vi "Write Section.vi"(8 "error in (no error)":errorcluster, 9 "Section Data":variant, 10 "Section Name":string, 11 "Configuration File in":refnum<class "Configuration File.lvclass">) -> (0 "error out":errorcluster, 3 "Configuration File out":refnum<class "Configuration File.lvclass">)   [LabVIEW 2019, in "Configuration File.lvlib" / "Configuration File.lvclass"]
doc: "This VI writes the variant's attributes in the section specified."
uses:
  Configuration File.lvclass
  Configuration File.lvclass/Configuration File.ctl
  <vilib>/Utility/config.llb/Write Key (String).vi
  <vilib>/Utility/config.llb/Write Key (Boolean).vi
  <vilib>/Utility/config.llb/Write Key (Double).vi
  <vilib>/Utility/config.llb/Write Key (U32).vi
  <vilib>/Utility/config.llb/Write Key (I32).vi
  <vilib>/Utility/config.llb/Write Key (Path).vi
  <vilib>/Utility/Data Type/NI_Data Type.lvlib
  <vilib>/Utility/config.llb/NI_LVConfig.lvlib
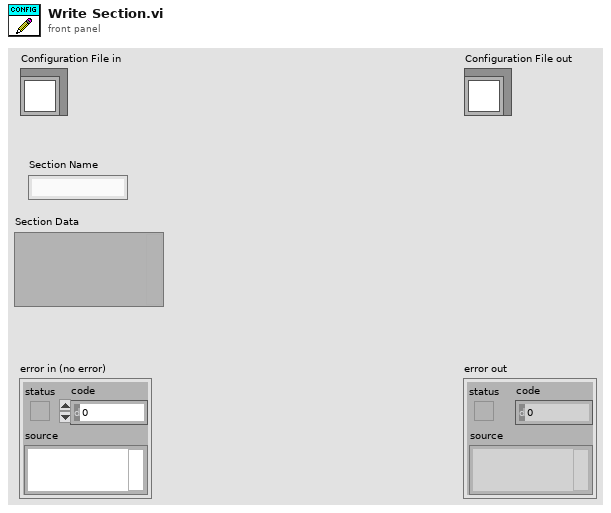
[diagram p1: front panel]
types:
  T1 = typedef "NI_LVConfig.lvlib/Config Data RefNum.ctl" = refnum<k1>
  T2 = typedef "NI_Data Type.lvlib/Data Type.ctl" = enum8{"Invalid Type", "Void", "I8", "I16", "I32", "I64", "U8", "U16", "U32", "U64", "Single Float", "Double Float", "Extended Float", "Single Complex", "Double Complex", "Extended Complex", "Enum U8", "Enum U16", "Enum U32", "Enum U64", "Single Float With Unit", "Double Float With Unit", "Extended Float With Unit", "Single Complex with Unit", "Double Complex with Unit", "Extended Complex with Unit", "Boolean", "String", "Path", "Picture", "Tag", "Array", "Cluster", "Variant", "LV Variant", "Waveform", "Timestamp", "Digital Waveform", "Digital Data", "ExpressData", "Refnum", "External Data", "VI", "Poly VI", "LabVIEW Class Instance", "Fixed Point", "Set Collection", "Map Collection"}
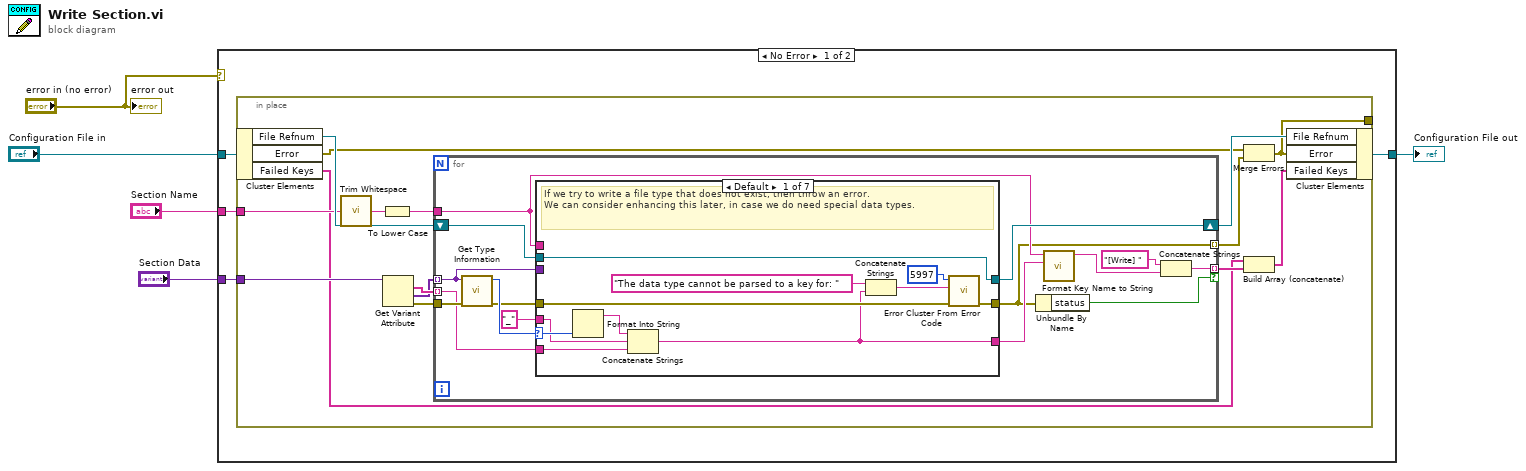
[diagram p0: block diagram]
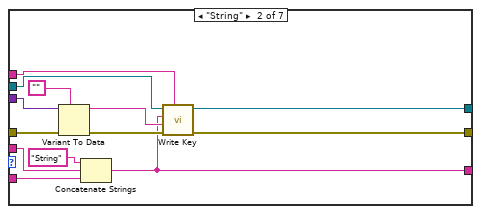
[diagram p2: hidden frame]
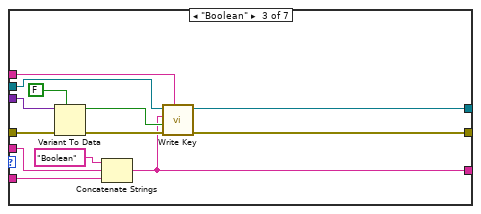
[diagram p3: hidden frame]
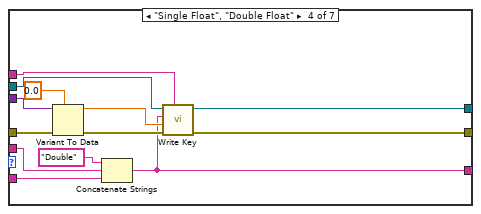
[diagram p4: hidden frame]
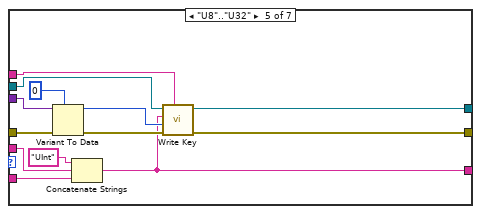
[diagram p5: hidden frame]
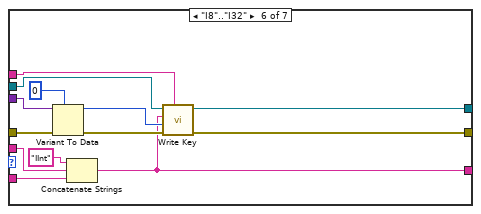
[diagram p6: hidden frame]
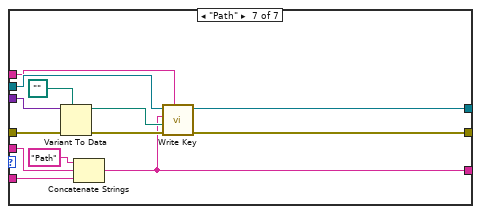
[diagram p7: hidden frame]
diagram:
  n1 = case shown="No Error" "error in (no error)" {
    tunnel: [w6 w129] -> w4
    tunnel: "Configuration File in" -> [w8 w129]
    tunnel: "Section Name" -> [w9 _]
    tunnel: "Section Data" -> [w7 _]
    frame No Error {
      n2 = in-place {
        in-place-border: w7 -> [w24]
        in-place-border: [w13] -> _
        in-place-border: w9 -> [w17]
        n3 = in-place-cluster #1(w8) -> ("File Refnum"=w18:T1, "Error"=w14:errorcluster, "Failed Keys"=w11:string[])
        n4 = call <vilib>:"Trim Whitespace.vi"("string"=w17) -> ("trimmed string"=w16:string)  [unwired: 1 in]
        n5 = To Lower Case(string=w16) -> (all lower case string=w15:string)
        n6 = Get Variant Attribute(Variant=w24) -> (names=w23:string[], values=w22:variant[], error out=w20:errorcluster)  [unwired: 3 in, 1 out]
        n7 = for {
          tunnel: w23 -> [w33] mode=indexing
          tunnel: w22 -> [w36] mode=indexing
          shift-right: [w34] -> w19
          shift-left: w18 -> [w35]
          tunnel: w15 -> [w31]
          tunnel: w20 -> [w39]
          tunnel: [w28] -> w21 mode=indexing
          tunnel: [w26] -> w12 mode=indexing if=w27
          n8 = call <vilib>:"Get Type Information.vi"("error in (no error)"=w39, "variant"=w36) -> ("error out"=w37:errorcluster, "type"=w38:T2)  [unwired: 5 in, 3 out]
          n9 = case shown="Default" w38 {
            selector: w38 -> [w46 _ _ _ _ _ _]
            tunnel: [w48 w63 w76 w89 w102 w115 w128] -> w28
            tunnel: w37 -> [w50 w55 w68 w81 w94 w107 w120]
            tunnel: w36 -> [_ w56 w69 w82 w95 w108 w121]
            tunnel: w35 -> [w49 w62 w75 w88 w101 w114 w127]
            tunnel: [w49 w61 w74 w87 w100 w113 w126] -> w34
            tunnel: w31 -> [_ w60 w73 w86 w99 w112 w125]
            tunnel: w33 -> [w44 w59 w72 w85 w98 w111 w124]
            tunnel: "_" ("string") -> [w45 w58 w71 w84 w97 w110 w123]
            tunnel: [w40 w51 w64 w77 w90 w103 w116] -> w30
            frame Default {
              # "If we try to write a file type that does not exist, then throw an error.\nWe can consider enhancing this later, in case we do need special data types."
              n10 = Format Into String(w46) -> (resulting string=w47:string)  [unwired: 3 in, 1 out]
              n11 = Concatenate Strings(w47, w45, w44) -> (w40:string)
              n12 = Concatenate Strings("The data type cannot be parsed to a key for: " ("error message (\"\")"), w40) -> (w41:string)
              n13 = call <vilib>:"Error Cluster From Error Code.vi"("error in (no error)"=w50, "error message (\"\")"=w41, "error code (0)"=5997) -> ("error out"=w48:errorcluster)  [unwired: 6 in]
            }
            frame "String" {
              n14 = Variant To Data(error in=w55, type="", Variant=w56) -> (data=w53:string, error out=w54:errorcluster)
              n15 = Concatenate Strings("String" ("string"), w58, w59) -> (w51:string)
              n16 = call-poly <vilib>:"Write Key.vi"("section"=w60, "error in (no error)"=w54, "value"=w53, "key"=w51, "refnum"=w62) -> ("error out"=w63:errorcluster, "refnum out"=w61:T1)  [unwired: 4 in, 1 out]
            }
            frame "Boolean" {
              n17 = Variant To Data(error in=w68, type=FALSE, Variant=w69) -> (data=w66:bool, error out=w67:errorcluster)
              n18 = Concatenate Strings("Boolean" ("string"), w71, w72) -> (w64:string)
              n19 = call-poly <vilib>:"Write Key.vi"("section"=w73, "error in (no error)"=w67, "value"=w66, "key"=w64, "refnum"=w75) -> ("error out"=w76:errorcluster, "refnum out"=w74:T1)  [unwired: 4 in, 1 out]
            }
            frame "Single Float", "Double Float" {
              n20 = Variant To Data(error in=w81, type=0.0, Variant=w82) -> (data=w79:dbl, error out=w80:errorcluster)
              n21 = Concatenate Strings("Double" ("string"), w84, w85) -> (w77:string)
              n22 = call-poly <vilib>:"Write Key.vi"("section"=w86, "error in (no error)"=w80, "value"=w79, "key"=w77, "refnum"=w88) -> ("error out"=w89:errorcluster, "refnum out"=w87:T1)  [unwired: 4 in, 1 out]
            }
            frame "U8".."U32" {
              n23 = Variant To Data(error in=w94, type=u32 0, Variant=w95) -> (data=w92:u32, error out=w93:errorcluster)
              n24 = Concatenate Strings("UInt" ("string"), w97, w98) -> (w90:string)
              n25 = call-poly <vilib>:"Write Key.vi"("section"=w99, "error in (no error)"=w93, "value"=w92, "key"=w90, "refnum"=w101) -> ("error out"=w102:errorcluster, "refnum out"=w100:T1)  [unwired: 4 in, 1 out]
            }
            frame "I8".."I32" {
              n26 = Variant To Data(error in=w107, type=0, Variant=w108) -> (data=w105:i32, error out=w106:errorcluster)
              n27 = Concatenate Strings("IInt" ("string"), w110, w111) -> (w103:string)
              n28 = call-poly <vilib>:"Write Key.vi"("section"=w112, "error in (no error)"=w106, "value"=w105, "key"=w103, "refnum"=w114) -> ("error out"=w115:errorcluster, "refnum out"=w113:T1)  [unwired: 4 in, 1 out]
            }
            frame "Path" {
              n29 = Variant To Data(error in=w120, type=path "", Variant=w121) -> (data=w118:path, error out=w119:errorcluster)
              n30 = Concatenate Strings("Path" ("string"), w123, w124) -> (w116:string)
              n31 = call-poly <vilib>:"Write Key.vi"("section"=w125, "error in (no error)"=w119, "value"=w118, "key"=w116, "refnum"=w127) -> ("error out"=w128:errorcluster, "refnum out"=w126:T1)  [unwired: 4 in, 1 out]
            }
          }
          n32 = Unbundle By Name(w28) -> ("status"=w27:bool)
          n33 = call "Format Key Name to String.vi"("Key"=w30, "Section"=w31) -> ("String out"=w29:string)  [unwired: 9 in]
          n34 = Concatenate Strings("[Write] " ("string"), w29) -> (w26:string)
        }
        n35 = Merge Errors(w14, w21) -> (w13:errorcluster)
        n36 = Build Array (concatenate)(w11, w12) -> (w10:string[])
        n37 = in-place-cluster #1("File Refnum"=w19, "Error"=w13, "Failed Keys"=w10) -> (w6:refnum<class "Configuration File.lvclass">)
      }
    }
    frame Error {
    }
  }
  "Configuration File out" <- w4
  "error out" <- "error in (no error)"
